vi "SetTargetPosition.vi"(0 "handle in":i32, 1 "UnitAddress(0)":u16, 2 "MotNr(0)":u8, 5 "error in":errorcluster, 7 "TargetPosition(0)":u8) -> (14 "handle out":i32, 19 "error out":errorcluster)   [LabVIEW 2014, in "Sixpack - Driver.lvlib"]
doc: "Verändert die Zielposition. Kann z.B. auch zur Verkürzung / Verlängerung einer Fahrrampe verwendet werden. Die Änderung der Zielposition und Fahrt auf das neue Ziel findet sofort statt, wenn der Motor aktiv ist. Bei stehendem Motor erfolgt eine Speicherung der Zielposition, es wird jedoch keine Motorbewegung ausgelöst.\n\nCMD $26\nMotorNr (0...5)\nTargetPosition"
uses:
  Sixpack - Driver.lvlib
  DLL/PackDLL.dll
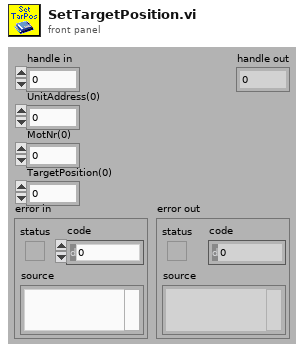
[diagram p1: front panel]
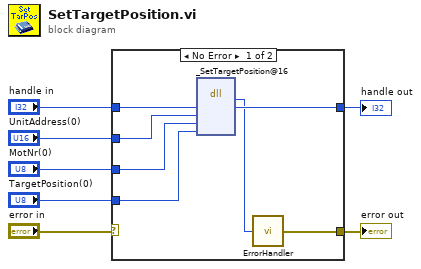
[diagram p0: block diagram]
diagram:
  n1 = case shown="No Error" "error in" {
    selector: "error in" -> [_ w15]
    tunnel: [w14 w16] -> w7
    tunnel: "handle in" -> [w13 w16]
    tunnel: "UnitAddress(0)" -> [w12 _]
    tunnel: "MotNr(0)" -> [w11 _]
    tunnel: "TargetPosition(0)" -> [w10 _]
    tunnel: [w8 w15] -> w2
    frame No Error {
      n2 = dll-call lib="D:/CS-Source/LV2014/GPL/instr.lib/SixPack/PackDLL/DLL/PackDLL.dll" fn="_SetTargetPosition@16" label="SetTargetPosition"("HANDLE"=w13, "UnitAddress"=w12, "MotNr"=w11, "TargetPosition"=w10) -> ("BOOLEAN"=w9:i8, "HANDLE"=w14:i32)  [unwired: 6 in, 2 out]
      n3 = call "ErrorHandler.vi"("BOOLEAN"=w9) -> ("error out"=w8:errorcluster)
    }
    frame Error {
    }
  }
  "handle out" <- w7
  "error out" <- w2
